vi "Load Action.vi"(8 "error in (no error)":errorcluster, 11 "Device in":refnum<class "Device.lvclass">) -> (0 "error out":errorcluster, 3 "Device out":refnum<class "Device.lvclass">)   [LabVIEW 2020, in "Device.lvlib" / "Device.lvclass"]
uses:
  Device.lvclass
  <vilib>/Utility/config.llb/NI_LVConfig.lvlib
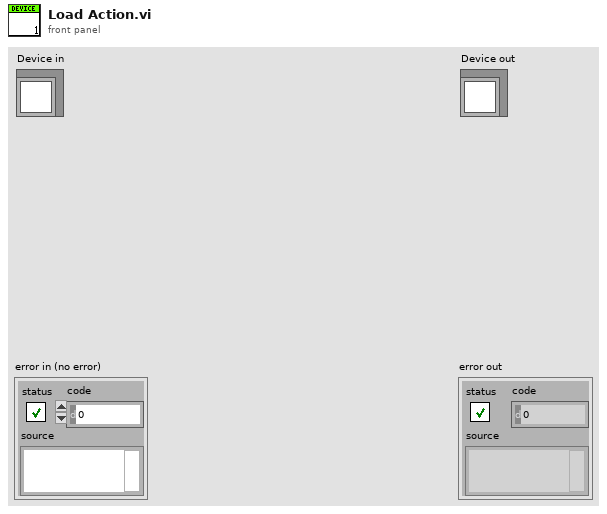
[diagram p1: front panel]
types:
  T1 = typedef "NI_LVConfig.lvlib/Config Data RefNum.ctl" = refnum<k1>
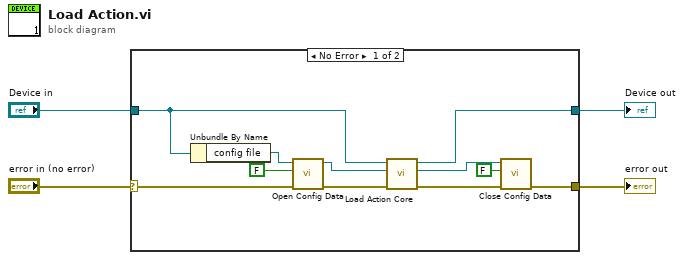
[diagram p0: block diagram]
diagram:
  n1 = case shown="No Error" "error in (no error)" {
    selector: "error in (no error)" -> [w15 w17]
    tunnel: [w6 w17] -> w3
    tunnel: [w9 w16] -> w1
    tunnel: "Device in" -> [w10 w16]
    frame No Error {
      n2 = Unbundle By Name(w10) -> ("config file"=w14:path)
      n3 = call <vilib>:"Open Config Data.vi"("error in (no error)"=w15, "create file if necessary (T)"=FALSE, "configuration file path"=w14) -> ("error out"=w12:errorcluster, "refnum"=w11:T1)  [unwired: 6 in, 1 out]
      n4 = call-dynamic "Load Action Core.vi"("error in (no error)"=w12, "config file in"=w11, "Device in"=w10) -> ("error out"=w8:errorcluster, "config file out"=w7:T1, "Device out"=w9:refnum<class "Device.lvclass">)  [unwired: 6 in]
      n5 = call <vilib>:"Close Config Data.vi"("error in (no error)"=w8, "write file if changed (T)"=FALSE, "refnum"=w7) -> ("error out"=w6:errorcluster)  [unwired: 7 in, 1 out]
    }
    frame Error {
    }
  }
  "error out" <- w3
  "Device out" <- w1
